vi "sandbox.vi"() -> ()   [LabVIEW 2016]
panel:
  out "unsigned byte array":u8[](array[numeric]) format="%x"
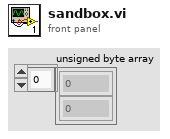
[diagram p1: front panel]
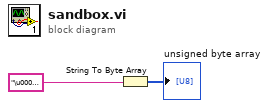
[diagram p0: block diagram]
diagram:
  n1 = String To Byte Array(string="\u0000\u0004") -> (unsigned byte array=→"unsigned byte array":u8[])
